vi "Skip_If Sd_Error_Below.vi"(0 "String to Search":string, 1 "Simulate/Run":T1, 2 "Measurement setup Applied?":bool, 3 "Row Number":i32, 5 "Measurement Setup File":string) -> (4 "Check for Skip?":bool, 6 "Error String":string, 7 "Instrument Code Name":string, 8 "Sd Error Theshold value":dbl, 9 "Minimum Measurement time (Sec)":dbl=6.0 format="%.2f")   [LabVIEW 2020]
uses:
  Controls/User_Specific_mode.ctl
  Globals/Extra_Commands_Global.vi
  Globals/Meas_global.vi
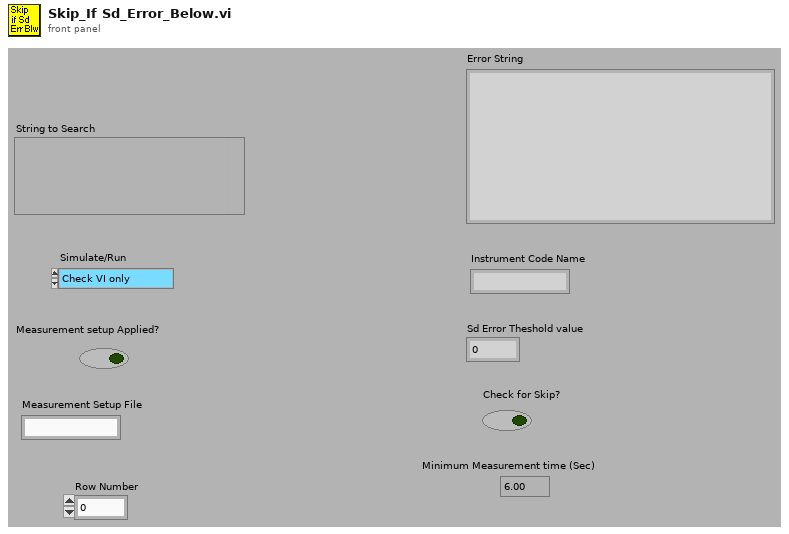
[diagram p1: front panel]
types:
  T1 = typedef "User_Specific_mode.ctl" = enum16{"Check VI only", "Run VI"}
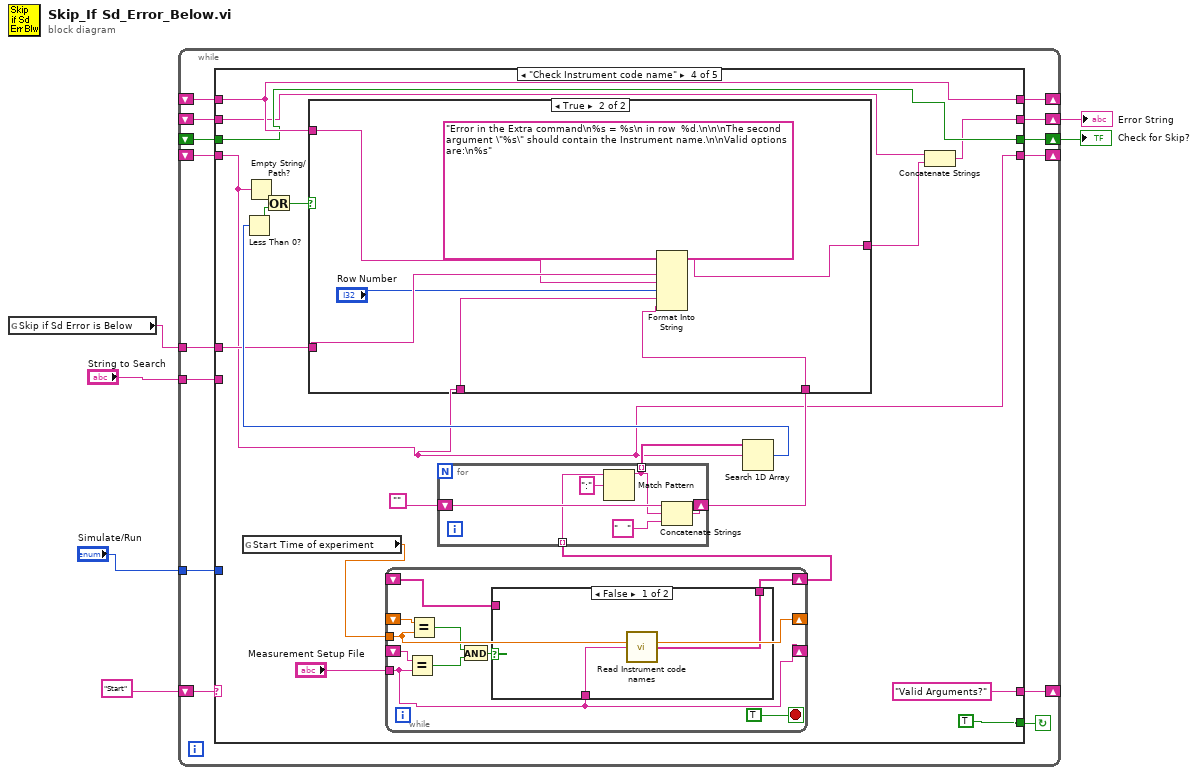
[diagram p0: block diagram]
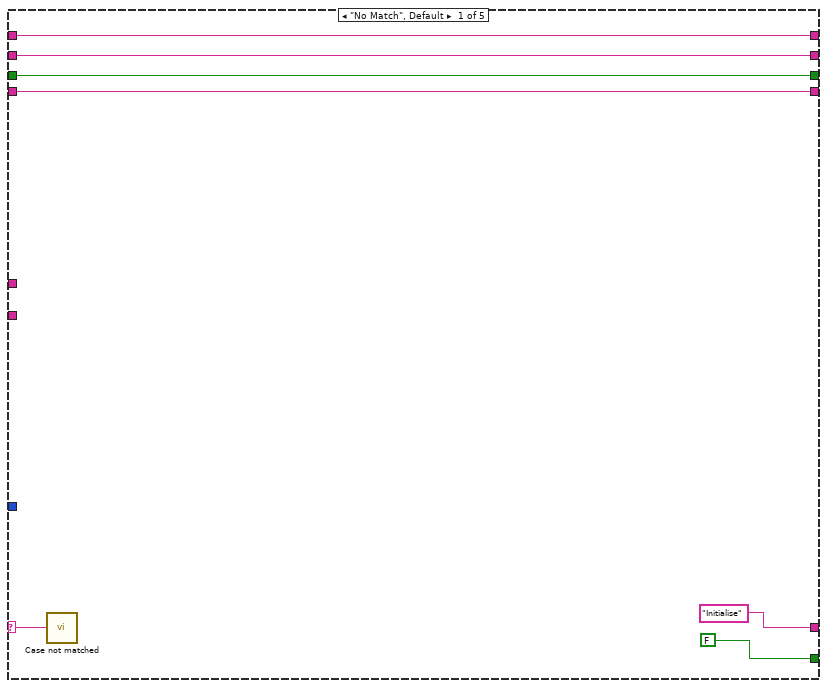
[diagram p2: hidden frame]
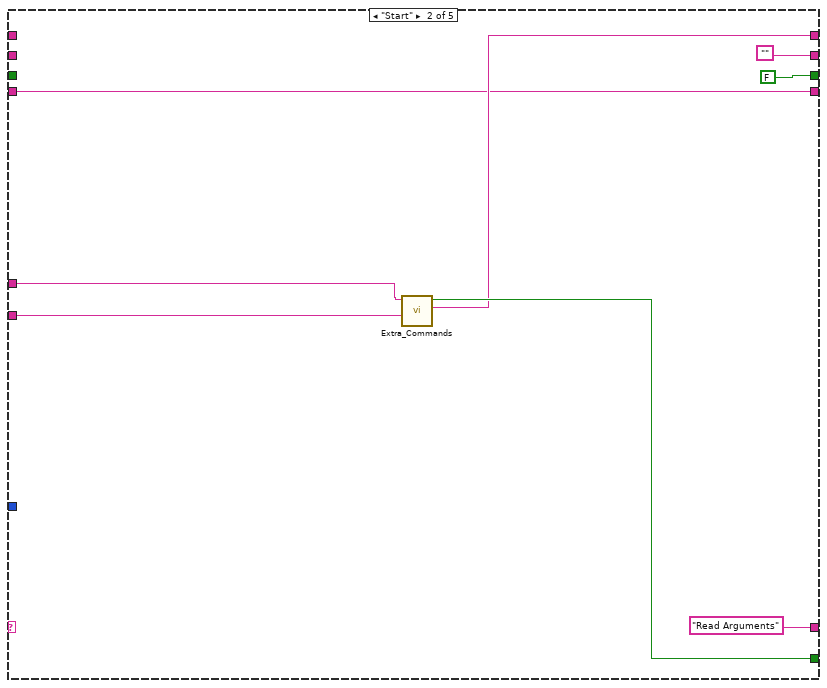
[diagram p3: hidden frame]
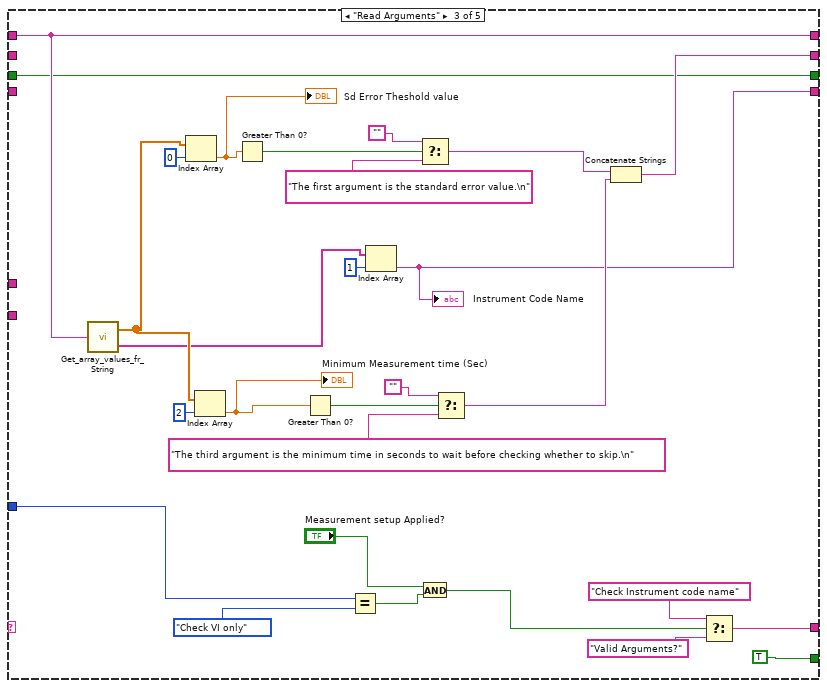
[diagram p4: hidden frame]
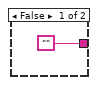
[diagram p6: hidden frame]
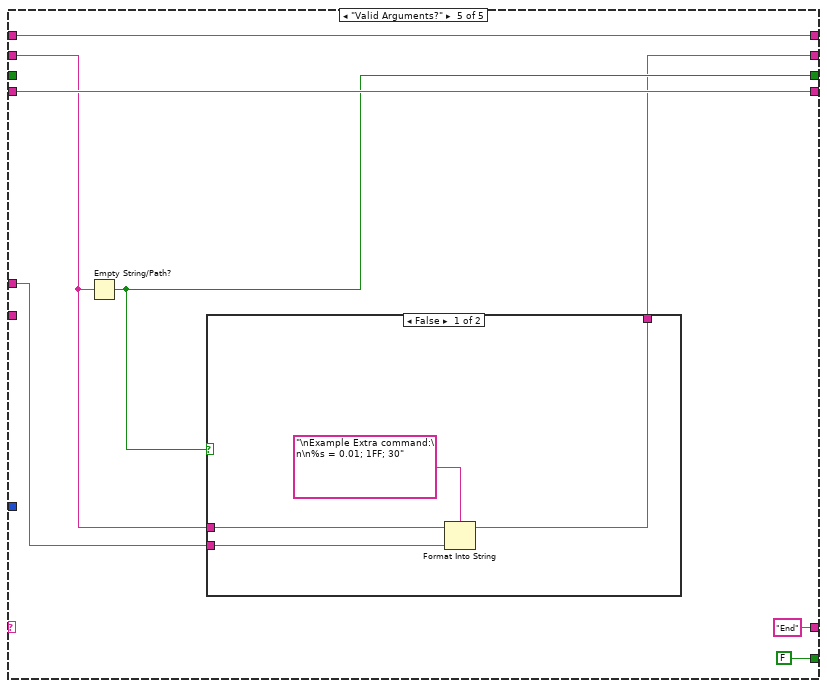
[diagram p7: hidden frame]
diagram:
  n1 = global read "Extra_Commands_Global.vi" "Skip if Sd Error is Below"() -> (w2:string)
  n2 = while {
    shift-left: "Start" -> [w18]
    shift-right: [w19] -> _
    tunnel: "String to Search" -> [w17]
    shift-right: [w16] -> _
    shift-left: _ -> [w13]
    shift-right: [w14] -> w4
    shift-left: _ -> [w12]
    shift-right: [w15] -> w3
    shift-left: _ -> [w11]
    tunnel: w2 -> [w10]
    shift-right: [w8] -> _
    shift-left: _ -> [w9]
    tunnel: "Simulate/Run" -> [w7]
    stop <- w20 continue-if-true
    n3 = case shown="\"Check Instrument code name\"" w18 {
      selector: w18 -> [w21 _ _ _ _]
      tunnel: [FALSE w33 TRUE TRUE FALSE ("Command Found")] -> w20
      tunnel: ["Initialise" "Read Arguments" w49 "Valid Arguments?" "End"] -> w19
      tunnel: w17 -> [_ w34 _ _ _]
      tunnel: [w25 w32 w47 w76 w117] -> w16
      tunnel: [w23 FALSE w40 w75 w113] -> w15
      tunnel: [w24 "" w41 w71 w110] -> w14
      tunnel: w13 -> [w25 _ w47 w76 w117]
      tunnel: w12 -> [w24 _ _ w73 w111]
      tunnel: w11 -> [w23 _ w40 w75 _]
      tunnel: w10 -> [_ w29 _ w77 w112]
      tunnel: w9 -> [w22 w28 _ w68 w116]
      tunnel: [w22 w28 w37 w68 w116] -> w8
      tunnel: w7 -> [_ _ w45 _ _]
      frame "No Match", Default {
        n4 = call "Case not matched.vi"("Case Name not Matched"=w21) -> ()
      }
      frame "Start" {
        n5 = call "Extra_Commands.vi"("String to Search"=w34, "Command"=w29) -> ("String Value"=w32:string, "Command Found"=w33:bool)  [unwired: 1 in, 3 out]
      }
      frame "Read Arguments" {
        n6 = call "Get_array_values_fr_String.vi"("String Value"=w47) -> ("Numeric Array"=w56:dbl[], "String array"=w52:string[])
        n7 = Index Array(array=w56, index=0) -> (element=w38:dbl)
        "Sd Error Theshold value" <- w38
        n8 = Index Array(array=w56, index=2) -> (element=w39:dbl)
        "Minimum Measurement time (Sec)" <- w39
        n9 = Greater Than 0?(x=w38) -> (x > 0?=w59:bool)
        n10 = Greater Than 0?(x=w39) -> (x > 0?=w53:bool)
        n11 = Equal?(x=w45, y=User_Specific_mode."Check VI only" ("Simulate/Run")) -> (x = y?=w44:bool)
        n12 = Index Array(array=w52, index=1) -> (element=w37:string)
        "Instrument Code Name" <- w37
        n13 = Select(t="", s=w59, f="The first argument is the standard error value.\n") -> (s? t:f=w51:string)
        n14 = And(x="Measurement setup Applied?", y=w44) -> (x .and. y?=w42:bool)
        n15 = Select(t="", s=w53, f="The third argument is the minimum time in seconds to wait before checking whether to skip.\n") -> (s? t:f=w50:string)
        n16 = Concatenate Strings(w51, w50) -> (w41:string)
        n17 = Select(t="Check Instrument code name", s=w42, f="Valid Arguments?") -> (s? t:f=w49:string)
      }
      frame "Check Instrument code name" {
        n18 = global read "Meas_global.vi" "Start Time of experiment"() -> (w64:dbl)
        n19 = Empty String/Path?(string/path=w68) -> (empty?=w69:bool)
        n20 = while {
          shift-right: [w91] -> w65
          shift-left: _ -> [w90]
          shift-right: [w88] -> _
          shift-left: _ -> [w92]
          tunnel: "Measurement Setup File" -> [w88]
          shift-right: [w86] -> _
          shift-left: _ -> [w87]
          tunnel: w64 -> [w86]
          stop <- TRUE stop-if-true
          n21 = Equal?(x=w92, y=w88) -> (x = y?=w84:bool)
          n22 = Equal?(x=w87, y=w86) -> (x = y?=w85:bool)
          n23 = And(x=w85, y=w84) -> (x .and. y?=w83:bool)
          n24 = case shown="False" w83 {
            tunnel: [w93 w95] -> w91
            tunnel: w90 -> [_ w95]
            tunnel: w88 -> [w94 _]
            frame False {
              n25 = call "Read Instrument code names.vi"("Measurement Setup File"=w94) -> ("List of Code Names"=w93:string[])
            }
            frame True {
            }
          }
        }
        n26 = for {
          tunnel: [w107] -> w81 mode=indexing
          shift-right: [w106] -> w78
          shift-left: "" -> [w108]
          tunnel: w65 -> [w104] mode=indexing
          n27 = Match Pattern(string=w104, regular expression=":") -> (before substring=w107:string)  [unwired: 4 out]
          n28 = Concatenate Strings(w108, w107, "   " ("string")) -> (w106:string)
        }
        n29 = Search 1D Array(1D array=w81, element=w68) -> (index of element=w79:i32)  [unwired: 1 out]
        n30 = Less Than 0?(x=w79) -> (x < 0?=w70:bool)
        n31 = Or(x=w69, y=w70) -> (x .or. y?=w67:bool)
        n32 = case shown="True" w67 {
          tunnel: w78 -> [_ w100]
          tunnel: w77 -> [_ w102]
          tunnel: w76 -> [_ w97]
          tunnel: w68 -> [_ w101]
          tunnel: ["" w99] -> w72
          frame False {
          }
          frame True {
            n33 = Format Into String(format string="Error in the Extra command\n%s = %s\n in row  %d.\n\n\nThe second argument \"%s\" should contain the Instrument name.\n\nValid options are:\n%s" ("f"), w102, w97, "Row Number", w101, w100) -> (resulting string=w99:string)  [unwired: 2 in, 1 out]
          }
        }
        n34 = Concatenate Strings(w73, w72) -> (w71:string)
      }
      frame "Valid Arguments?" {
        n35 = Empty String/Path?(string/path=w111) -> (empty?=w113:bool)
        n36 = case shown="False" w113 {
          tunnel: w112 -> [w120 _]
          tunnel: w111 -> [w119 w122]
          tunnel: [w118 w122] -> w110
          frame False {
            n37 = Format Into String(format string="\nExample Extra command:\n\n%s = 0.01; 1FF; 30", initial string=w119, w120) -> (resulting string=w118:string)  [unwired: 1 in, 1 out]
          }
          frame True {
          }
        }
      }
    }
  }
  "Error String" <- w4
  "Check for Skip?" <- w3
